vi "Configure Element.vi"(8 "error in (no error)":errorcluster, 9 "Crest Factor (3: CF3)":i32(ring)=3 items=["CF3"=3, "CF6"=6], 10 "Enable Independent Element (F: Disable)":bool, 11 "VISA resource name":refnum<visa-resource-name>) -> (0 "error out":errorcluster, 3 "VISA resource name out":refnum<visa-resource-name>)   [LabVIEW 2021, in "Yokogawa WT1800 Series.lvlib"]
doc: "Configures the element features."
uses:
  <instrlib>/Yokogawa WT1800 Series/Yokogawa WT1800 Series.lvlib
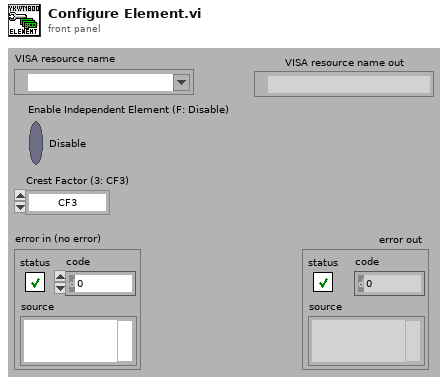
[diagram p1: front panel]
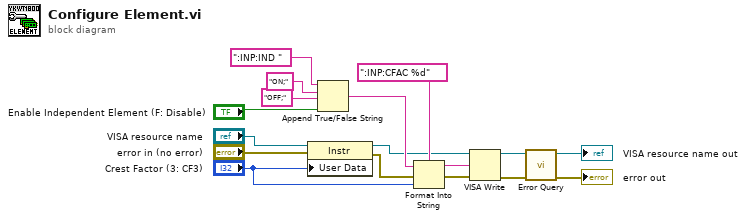
[diagram p0: block diagram]
diagram:
  n1 = property class="Instr"(reference="VISA resource name", error in="error in (no error)", "User Data"="Crest Factor (3: CF3)") -> (reference out=w4:refnum<visa-resource-name>, error out=w2:errorcluster)
  n2 = Append True/False String ("True/False 文字列を追加")(1:"Enable Independent Element (F: Disable)", 2:"OFF;", 3:"ON;", 4:":INP:IND ") -> (0:w6:string)
  n3 = Format Into String(format string=":INP:CFAC %d" ("形式文字列"), initial string=w6, error in=w2, "Crest Factor (3: CF3)") -> (resulting string=w8:string, error out=w7:errorcluster)
  n4 = VISA Write ("VISA書き込み")(VISA resource name=w4, write buffer=w8, error in (no error)=w7) -> (VISA resource name out=w15:refnum<visa-resource-name>, error out=w14:errorcluster)  [unwired: 1 out]
  n5 = call <instrlib>:"Error Query.vi"("error in (no error)"=w14, "VISA resource name"=w15) -> ("error out"=→"error out":errorcluster, "VISA resource name out"=→"VISA resource name out":refnum<visa-resource-name>)  [unwired: 6 in, 2 out]
